vi "Close VI.vi"(11 "VI in":refnum<vi>) -> ()   [LabVIEW 2020]
panel:
  out "error out":errorcluster
  in  "error in (no error)":errorcluster
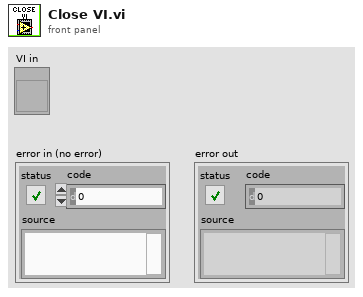
[diagram p1: front panel]
types:
  T1 = enum32{"Invalid", "Standard", "Closed", "Hidden", "Minimized", "Maximized"}
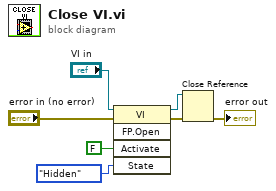
[diagram p0: block diagram]
diagram:
  n1 = invoke class="VI" method="FP.Open"(reference="VI in", error in="error in (no error)", "Activate"=FALSE ("Activate?"), "State"=T1."Hidden") -> (reference out=w6:refnum<vi>, error out=w5:errorcluster)  [unwired: 1 in, 3 out]
  n2 = Close Reference(reference=w6, error in (no error)=w5) -> (error out=→"error out":errorcluster)
